vi "Keyence_VS150.vi"(9 "Setting Value":string, 10 "Row No.":string, 11 "Coulumn No.":string) -> (3 "Inspection_Result":bool)   [LabVIEW 2024, in "Keyence_VS150.lvlib"]
doc: "This template is for the Queued Message Handler design pattern.\n\nThe Event Handling Loop generates messages based on user interface actions.\n\nThe Message Handling Loop processes messages generated by the Event Handling Loop, or by other messages. The messages are string values, so new messages can be added easily to the Message Cases case structure in the Message Handling Loop. Each message cluster can also provide an optional value for Message Data, which is a variant that can be converted to whatever message-specific data is required."
uses:
  Keyence_VS150.lvlib
  controls/UI Data.ctl
  Settings/support/Camera.ctl
  <userlib>/_OpenG.lib/array/array.llb/Search 1D Array (String)__ogtk.vi
  <vilib>/Utility/error.llb/Error Cluster From Error Code.vi
  <vilib>/ErrorRing/Error Ring.xnode
  Keysight_34461a/support/Message Queue/Message Queue.lvlib
  support/User Event - Stop/User Event - Stop.lvlib
  support/Message Queue/Message Queue.lvlib
  <userlib>/_OpenG.lib/string/string.llb/openg_string.lvlib
  Launcher/Launcher_DTU.lvlib
  <userlib>/_OpenG.lib/array/array.llb/openg_array.lvlib
  Settings/Setting_Screen.lvlib
panel:
  out "Saturation_Values 2":string
  out "transposed array":string[][](array[string])
  out "appended array":string[][](array[string])
  out "Saturation_Values":string[](array[string])
  in  "Row No. 2":string
  in  "Coulumn No. 2":string
  in  "Setting Value 2":string
  in  "Storage 2":string
  in  "Program No 2":string
  out "data 2":string
  out "Get Mode 2":string
  in  "Change_Program":bool
  out "RX/RY":string
  out "RX,RY":string
  out "status":bool
  in  "Trigger":bool
  in  "Total_Result":T1
  out "DTU 2":string[][](array[string])
  out "DTU1":string[][](array[string])
  out "DTU_Failed_Inspections_Array":string[](array[string])
  out "Fail":i32[](array[numeric])
  out "Inspection_names":string[](array[string])
  out "Result_Values":string[](array[string])
  out "DTU_Failed_Inspections":string
  in  "Config":string
  out "queue name 2":string
  out "queue name":string
  in  "ip address":string="169.254.73.187"
  in  "DUT":string
  out "Result Value":string[](array[string])
  out "Array of Strings":string[](array[string])
  out "data out":string
  out "data":string
  out "Get Mode":string
  in  "Program No":string
  in  "Storage":string
  out "Display <Replace Me>":string
  in  "Exit":bool
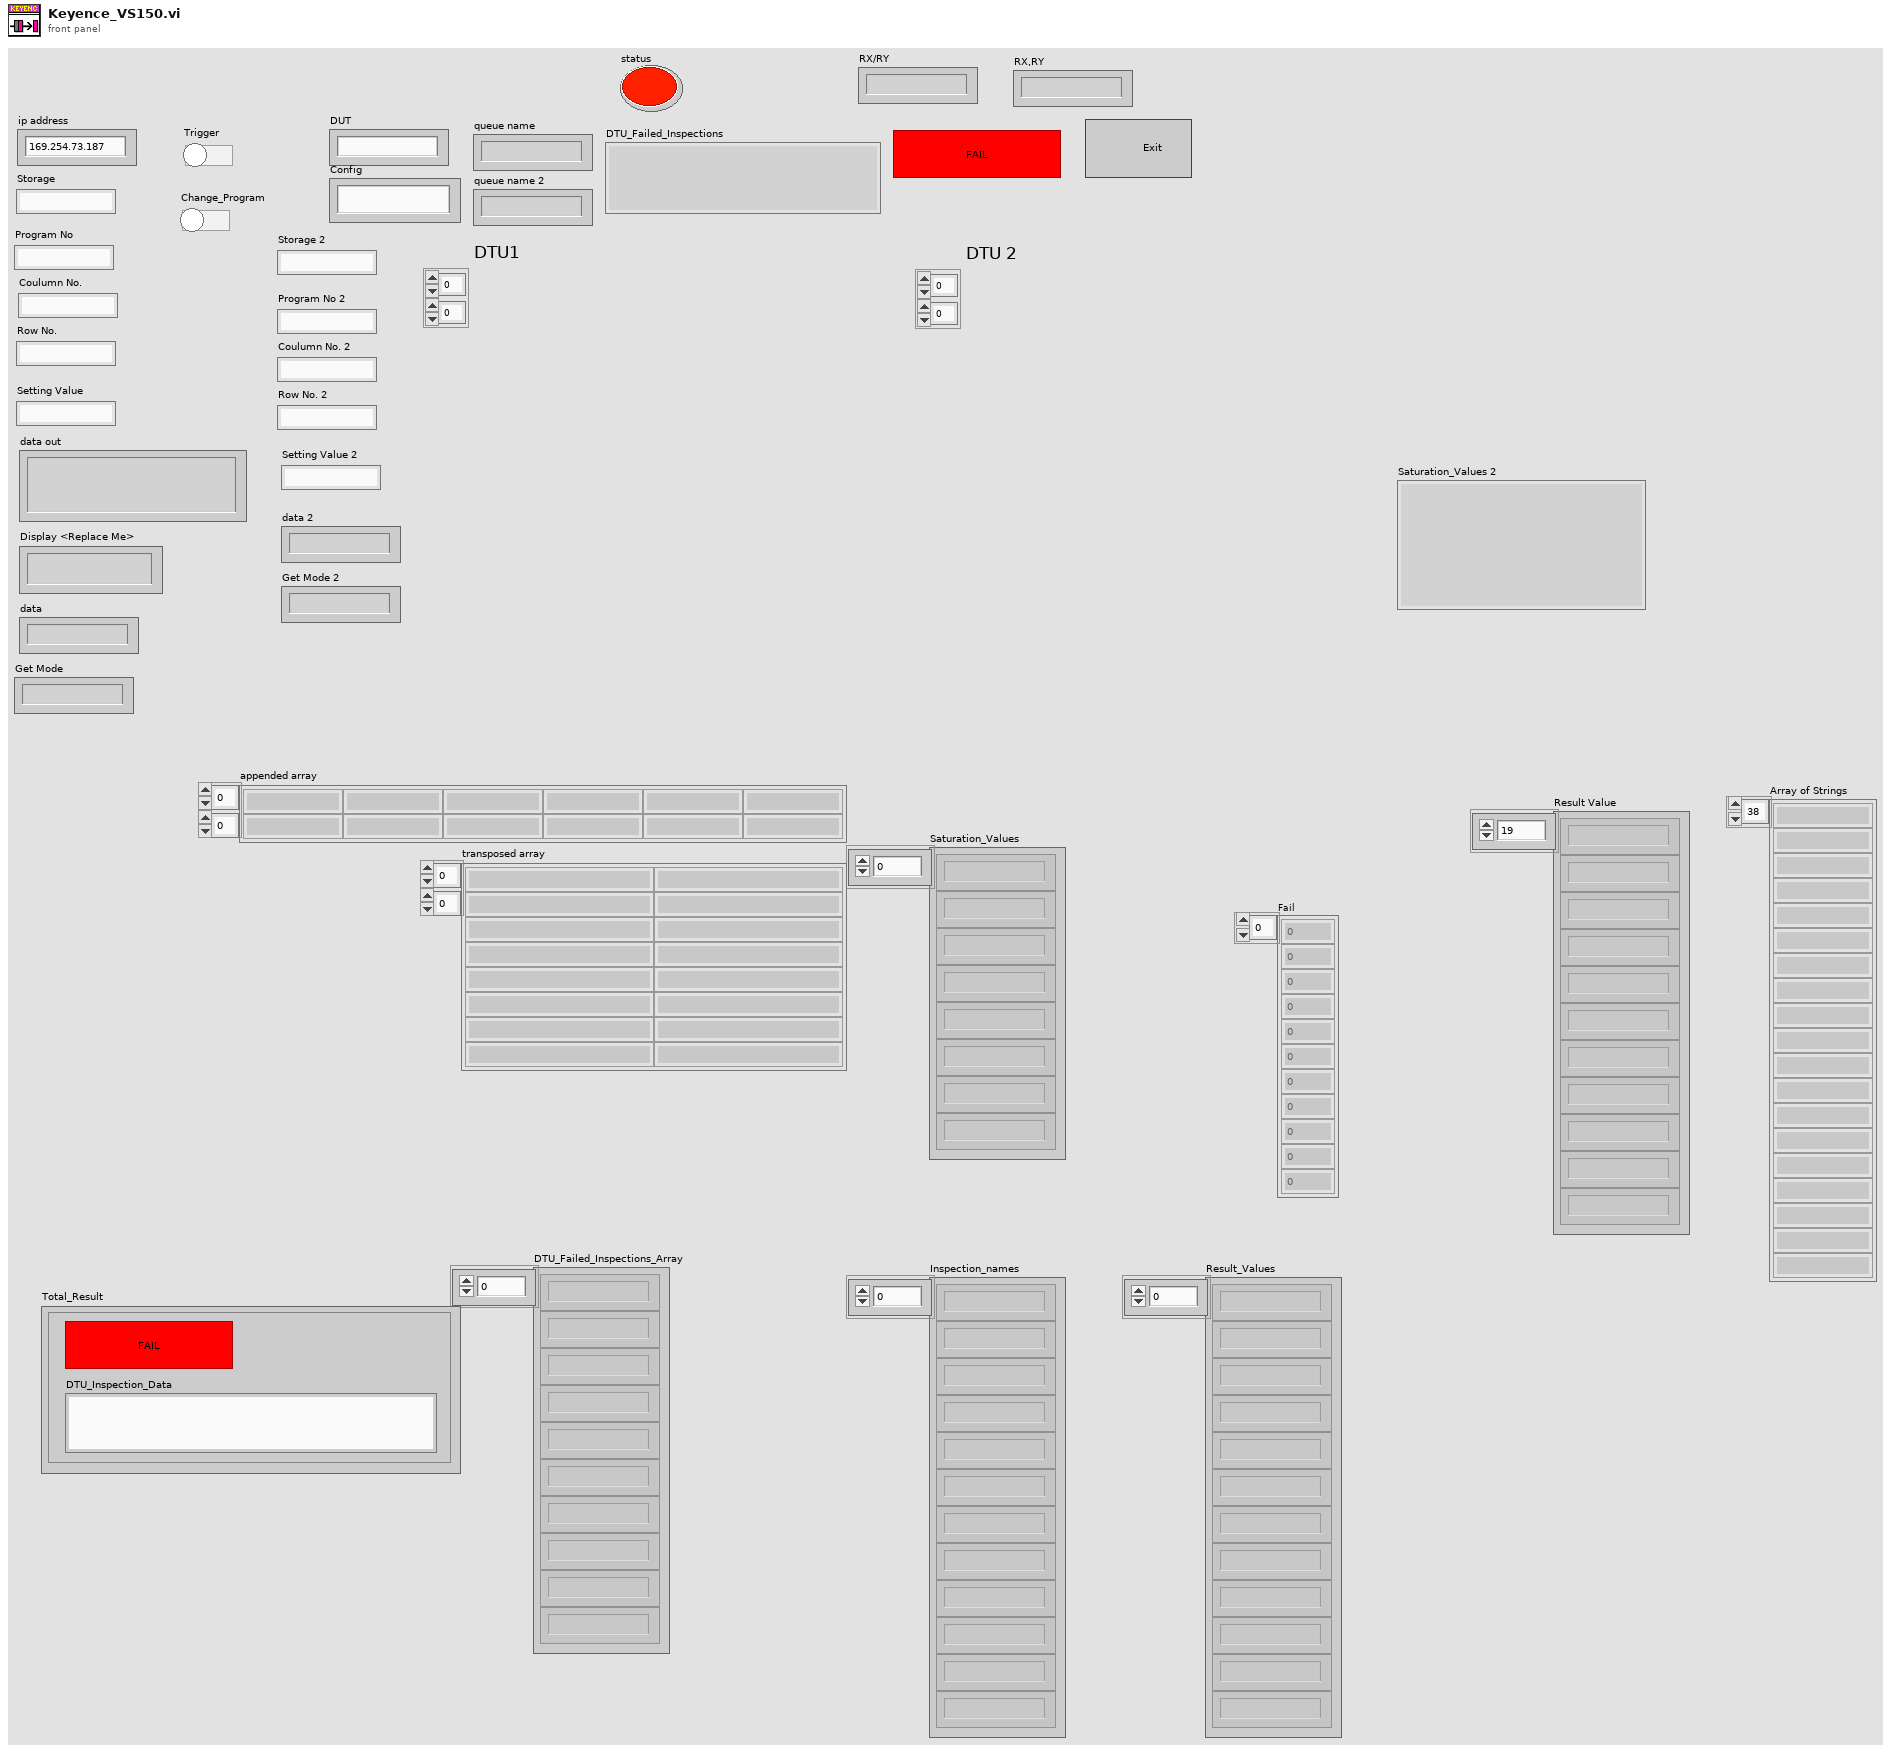
[diagram p1: front panel]
types:
  T1 = cluster{"Inspection_Result 2":bool, "DTU_Inspection_Data":string}
  T2 = typedef "Keyence_VS150.lvlib/UI Data.ctl" = cluster{"Boolean <Replace Me>":bool, "String <Replace Me>":string, "Numeric <Replace Me>":dbl, "Data Display Ref":refnum<vi>, "Exit Button Ref":refnum<vi>, "connection ID":refnum<k5>, "data out":string, "notifier out":refnum<notifier>, "DUT":string, "Config":string, "Keyence_VS150":refnum<queue>, "Result Value":string[], "Inspection_Result":bool, "Total_Result":cluster{"Inspection_Result 2":bool, "Inspection_Data":string}, "Camera":T3, "Camera_Program No":string, "DUT1":string, "DUT2":string, "Saturation_Values":string[]}
  T3 = typedef "Setting_Screen.lvlib/Camera.ctl" = cluster{"Trigger":bool, "Prog No.":string, "Delay":bool, "Delay time":dbl, "Storage":string, "Col no.":string, "Row no.":string}
  T4 = typedef "Keyence_VS150.lvlib/Message Queue.lvlib/All Message Queues.ctl" = cluster{"UI":refnum<queue>, "QSM":refnum<queue>}
  T5 = cluster{"Message":string, "Message Data":variant}
  T6 = enum16{"Read", "Write", "All_sections", "All_values", "Remove key&section"}
  T7 = cluster{"Status":string, "Free/inuse":bool, "Action":string}
  T8 = enum16{"Standard", "Buffered", "CRLF", "Immediate"}
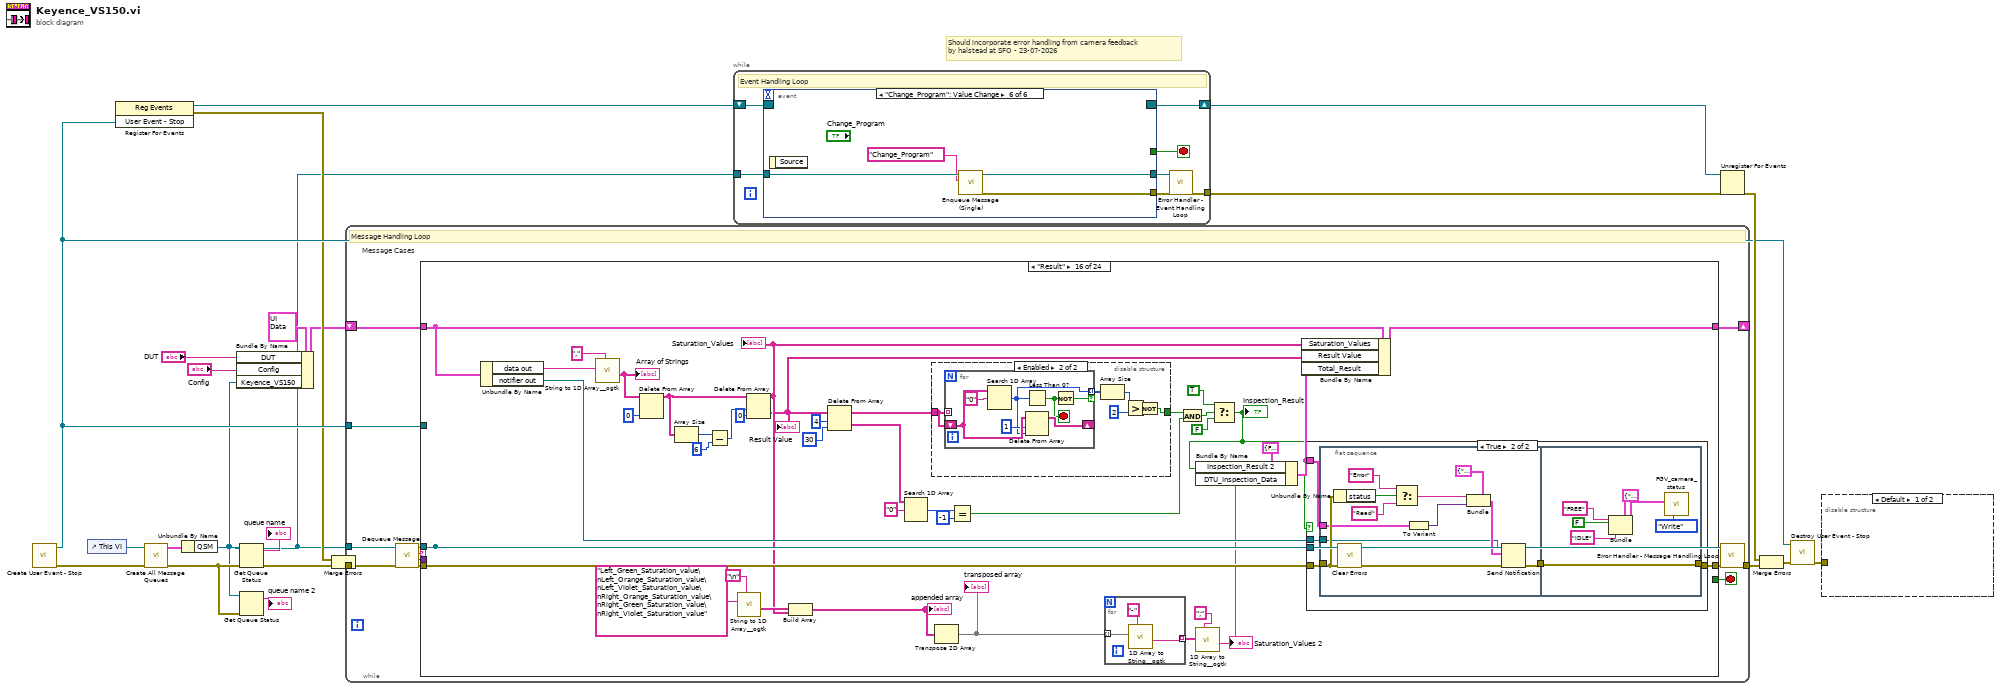
[diagram p0: block diagram]
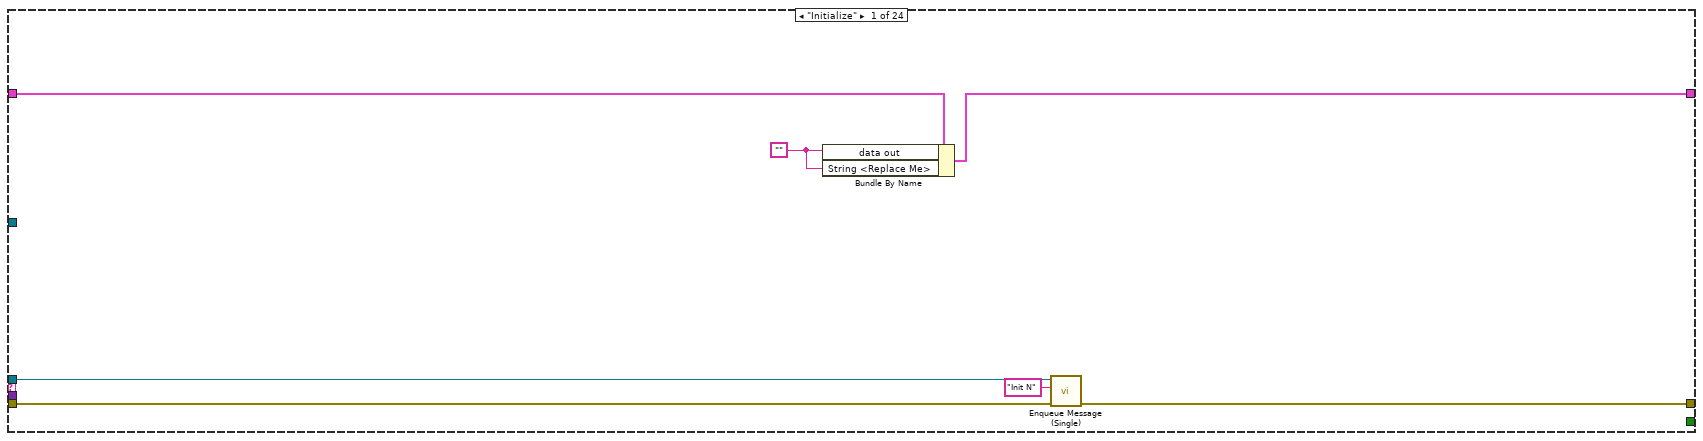
[diagram p2: hidden frame]
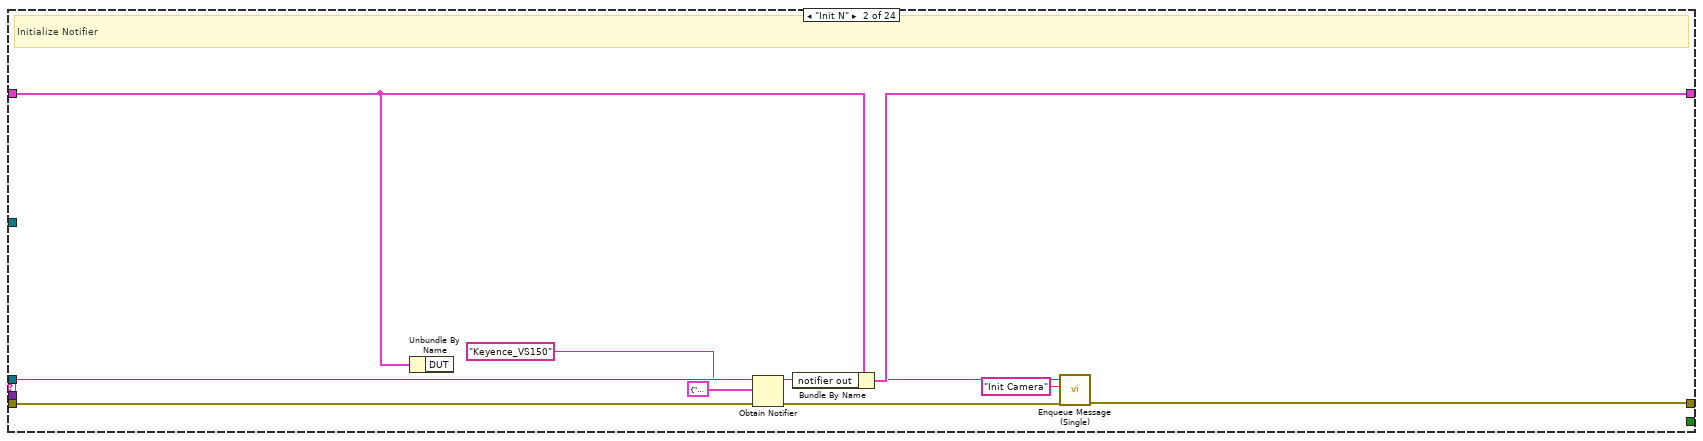
[diagram p3: hidden frame]
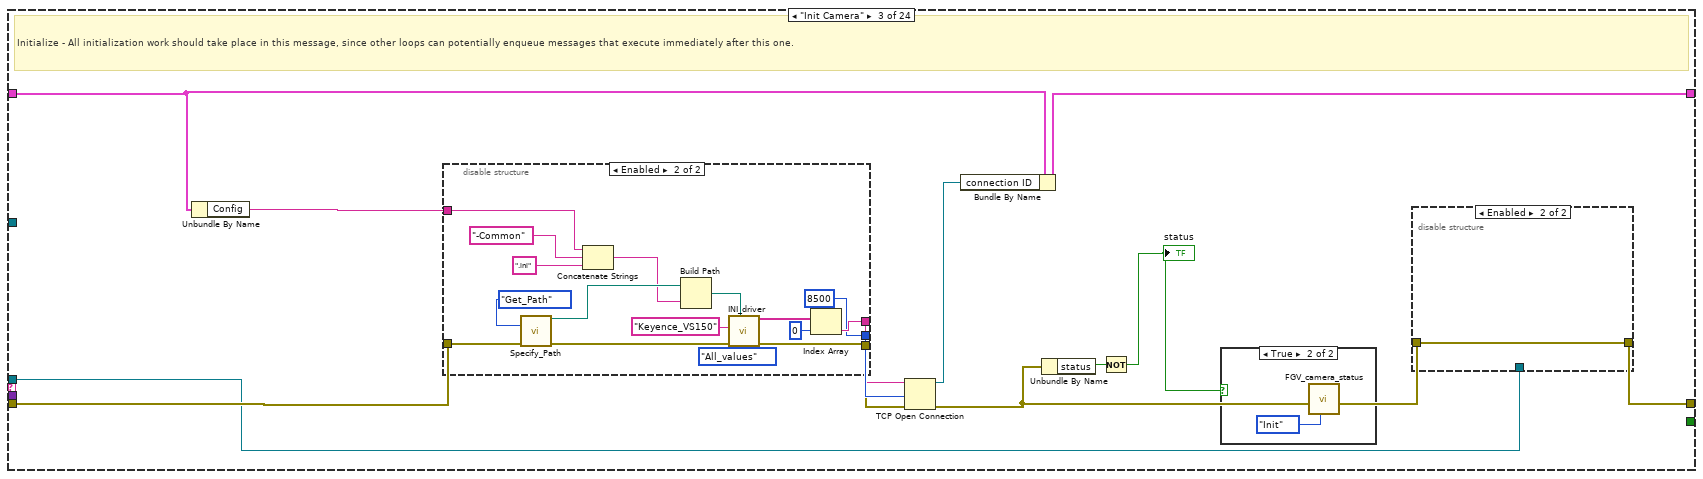
[diagram p4: hidden frame]
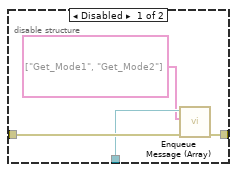
[diagram p5: hidden frame]
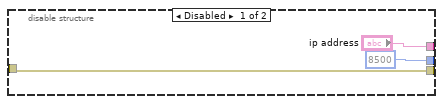
[diagram p7: hidden frame]
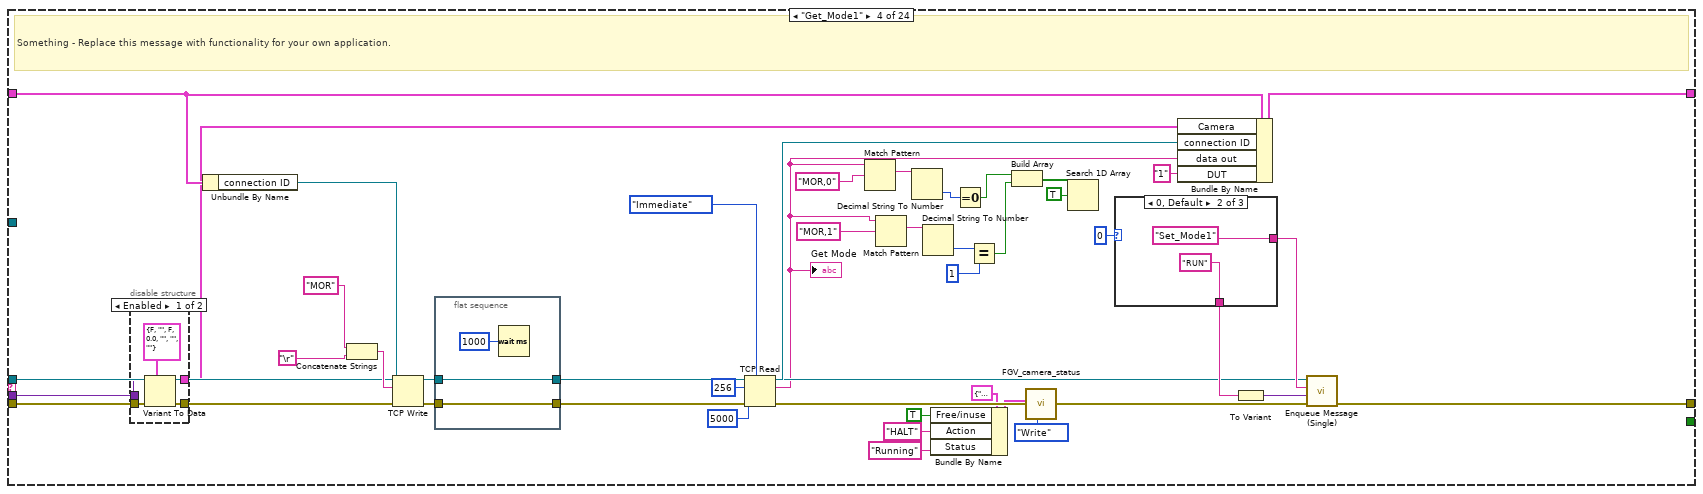
[diagram p8: hidden frame]
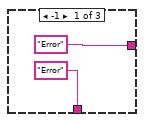
[diagram p10: hidden frame]
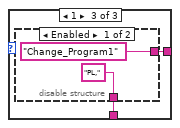
[diagram p11: hidden frame]
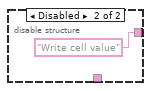
[diagram p12: hidden frame]
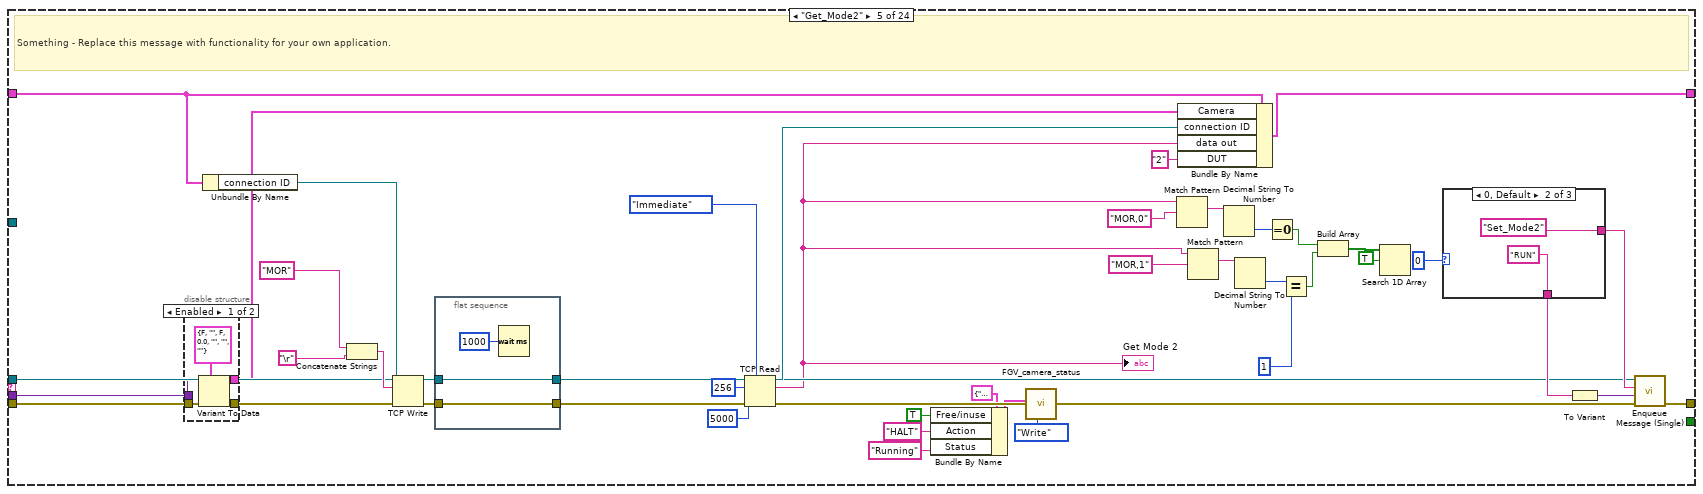
[diagram p13: hidden frame]
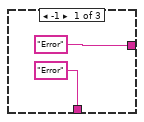
[diagram p15: hidden frame]
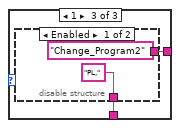
[diagram p16: hidden frame]
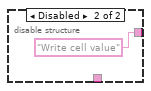
[diagram p17: hidden frame]
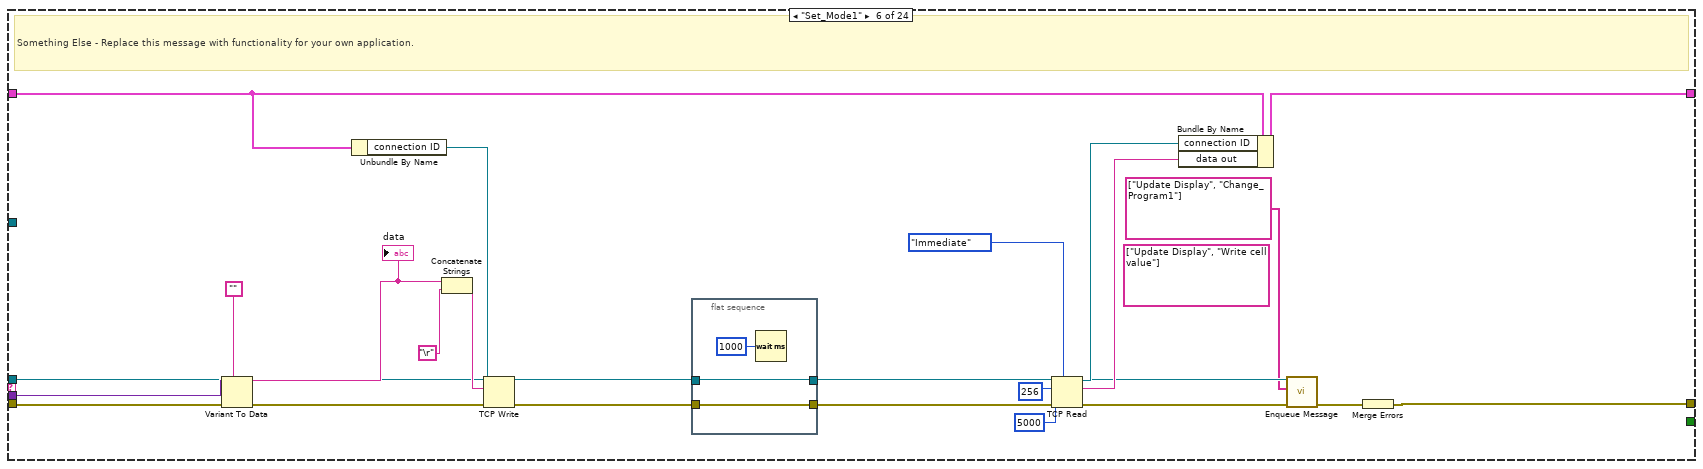
[diagram p18: hidden frame]
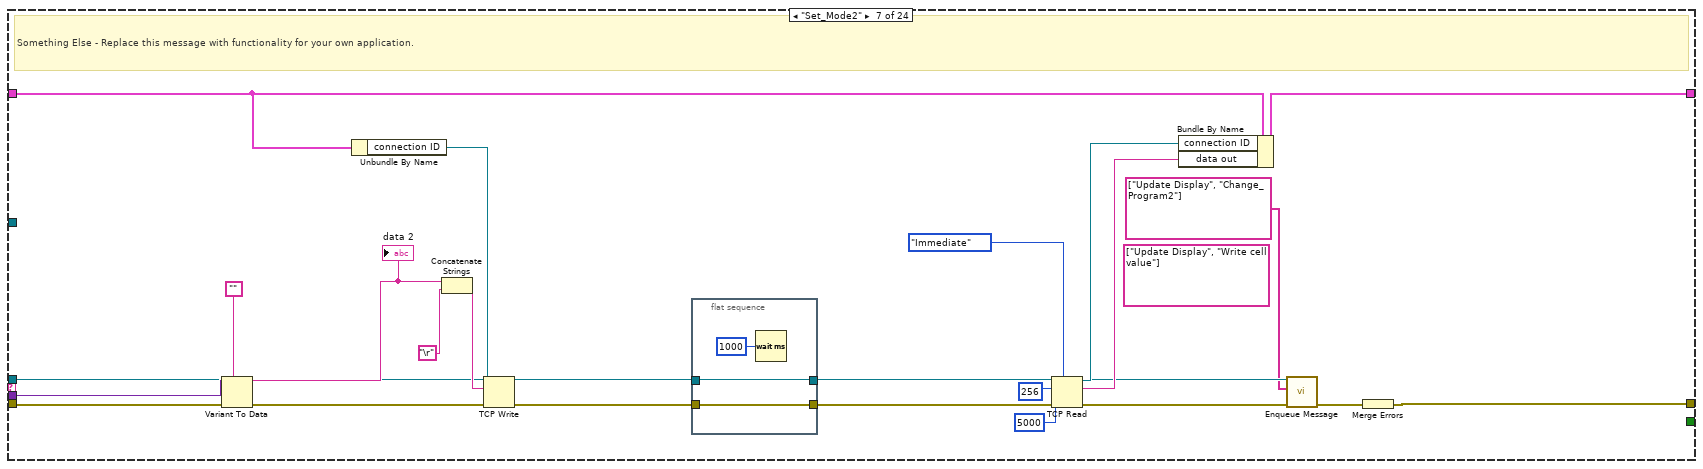
[diagram p19: hidden frame]
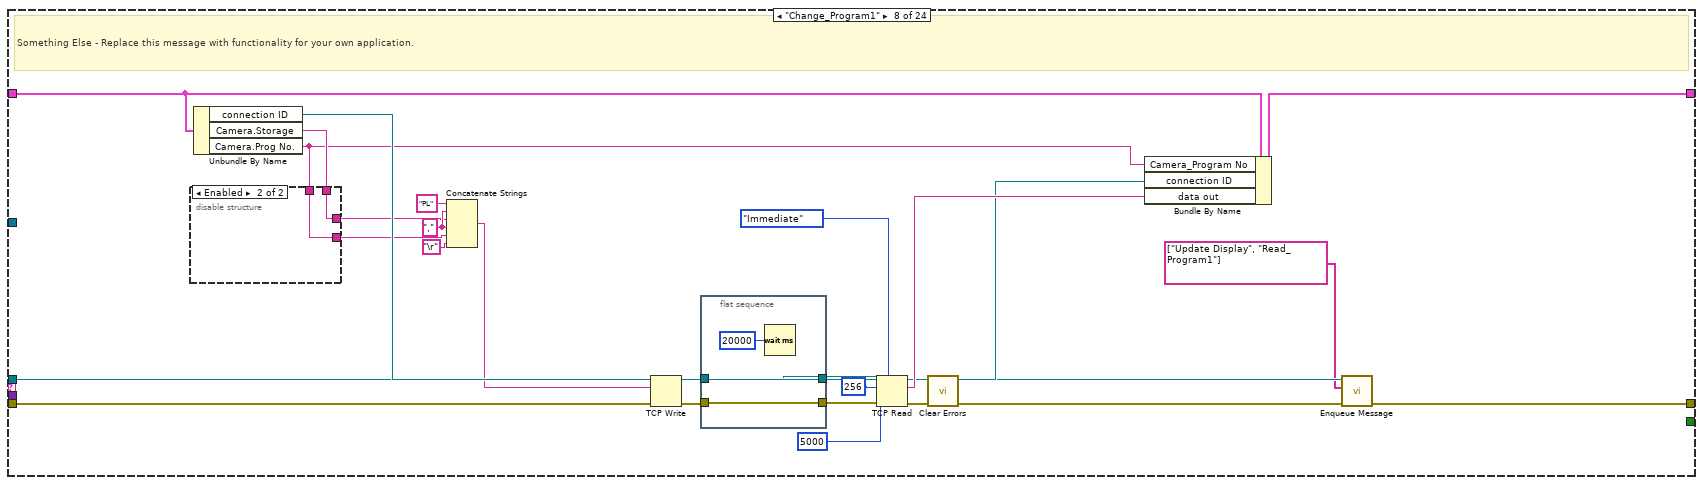
[diagram p20: hidden frame]
diagram:
  # "Should incorporate error handling from camera feedback\nby halstead at SFO - 23-07-2026"
  n1 = call "Create User Event - Stop.vi"() -> ("error out"=w21:errorcluster, "User Event - Stop"=w14:refnum<user-event>)  [unwired: 10 in]
  n2 = control-ref of="This VI"() -> (w9:refnum<vi>)
  n3 = register-events(w14) -> (reference out=w15:refnum<event-registration>, error out=w12:errorcluster)  [unwired: 2 in]
  n4 = call "Create All Message Queues.vi"("error in (no error)"=w21, "This VI"=w9) -> ("error out"=w3:errorcluster, "Message Queues out"=w23:T4)  [unwired: 8 in]
  n5 = Unbundle By Name(w23) -> ("QSM"=w1:refnum<queue>)
  n6 = Bundle By Name(cluster=T2 {"Boolean <Replace Me>"=FALSE, "String <Replace Me>"="", "Numeric <Replace Me>"=0.0, "Data Display Ref"=refnum, "Exit Button Ref"=refnum, "connection ID"=refnum, "data out"="", "notifier out"=refnum, "DUT"="", "Config"="", "Keyence_VS150"=refnum, "Result Value"=[], "Inspection_Result"=FALSE, "Total_Result"={"Inspection_Result 2"=FALSE, "Inspection_Data"=""}, "Camera"={"Trigger"=FALSE, "Prog No."="", "Delay"=FALSE, "Delay time"=0.0, "Storage"="", "Col no."="", "Row no."=""}, "Camera_Program No"="", "DUT1"="", "DUT2"="", "Saturation_Values"=[]} ("Data Cluster"), "DUT"="DUT", "Config"="Config", "Keyence_VS150"=w1) -> (w10:T2)
  n7 = Get Queue Status(queue=w1, error in (no error)=w3) -> (queue out=w5:refnum<queue>, queue name=→"queue name":string, error out=w4:errorcluster)  [unwired: 1 in, 5 out]
  n8 = Get Queue Status(queue=w1, error in (no error)=w3) -> (queue name=→"queue name 2":string)  [unwired: 1 in, 7 out]
  n9 = Merge Errors(w12, w4) -> (w13:errorcluster)
  n10 = while {
    tunnel: w5 -> [w27]
    shift-right: [w34] -> _
    shift-left: w10 -> [w35]
    tunnel: w14 -> [w32]
    tunnel: w13 -> [w31]
    tunnel: [w25] -> w22
    stop <- w33 stop-if-true
    # "Message Handling Loop"
    n11 = call "Dequeue Message.vi"("error in (no error)"=w31, "Message Queue"=w27) -> ("error out"=w30:errorcluster, "Message Data"=w28:variant, "Message"=w29:string, "dup Message Queue"=w26:refnum<queue>)  [unwired: 6 in]
    n12 = case "Message Cases" shown="\"Result\"" w29 {
      selector: w29 -> [_ _ _ _ _ _ _ _ _ _ _ _ _ _ _ _ _ _ _ _ _ _ _ w847]
      tunnel: w26 -> [w37 w45 w54 w116 w177 w219 w246 w284 w317 w338 w385 w452 w503 w547 w575 w637 _ _ _ _ _ w830 w846 _]
      tunnel: w30 -> [w39 w51 w60 w131 w192 w229 w256 w285 w318 w339 w386 w446 w497 w540 w568 w629 w706 w779 w807 w817 w822 w825 w838 _]
      tunnel: [w38 w47 w53 w102 w163 w236 w263 w292 w325 w344 w391 w453 w504 w549 w557 w639 w713 w778 w808 w811 w820 w831 w843 w848] -> w24
      tunnel: w35 -> [w42 w44 w59 w123 w184 w223 w250 w289 w322 w335 w382 w443 w494 w537 w566 w641 w712 w782 w806 w816 w821 w823 w837 w849]
      tunnel: [w40 w49 w64 w122 w183 w222 w249 w288 w321 w341 w388 w442 w493 w536 w565 w640 w712 w782 w806 w816 w821 w823 w837 w849] -> w34
      tunnel: [_ _ _ _ _ _ _ _ _ _ _ _ _ _ _ _ _ _ _ _ _ _ TRUE _] -> w33
      tunnel: w28 -> [_ _ _ w100 w161 w226 w253 _ _ _ _ _ _ _ _ _ _ _ _ w815 _ _ w839 _]
      tunnel: w32 -> [_ _ _ _ _ _ _ _ _ _ _ _ _ _ _ _ _ _ _ _ _ _ w842 _]
      frame "Initialize" {
        w41 = "" ("data out")
        n13 = Bundle By Name(cluster=w42, "data out"=w41, "String <Replace Me>"=w41) -> (w40:T2)
        n14 = call "Enqueue Message (Single).vi"("error in (no error)"=w39, "Message"="Init N", "Message Queue"=w37) -> ("error out"=w38:errorcluster)  [unwired: 7 in, 1 out]
      }
      frame "Init N" {
        # "Initialize Notifier"
        n15 = Unbundle By Name(w44) -> ()  [unwired: 1 out]
        n16 = Obtain Notifier(name (unnamed)="Keyence_VS150", notification data type=T5 {"Message"="", "Message Data"=variant} ("notification"), error in (no error)=w51) -> (notifier out=w50:refnum<notifier>, error out=w48:errorcluster)  [unwired: 1 in, 1 out]
        n17 = Bundle By Name(cluster=w44, "notifier out"=w50) -> (w49:T2)
        n18 = call "Enqueue Message (Single).vi"("error in (no error)"=w48, "Message"="Init Camera", "Message Queue"=w45) -> ("error out"=w47:errorcluster)  [unwired: 7 in, 1 out]
      }
      frame "Init Camera" {
        # "Initialize - All initialization work should take place in this message, since other loops can potentially enqueue messages that execute immediately after this one."
        n19 = Unbundle By Name(w59) -> ("Config"=w58:string)
        n20 = disable-structure shown="Enabled" {
          disable-tunnel: [u16 8500 ("remote port or service name") u16 8500 ("remote port or service name")] -> w65
          disable-tunnel: ["ip address" w77] -> w62
          disable-tunnel: [w72 w78] -> w61
          disable-tunnel: w60 -> [w72 w79]
          disable-tunnel: w58 -> [_ w76]
          frame Disabled {
          }
          frame Enabled {
            n21 = call "Specify_Path.vi"("Path_Enum"=enum16{"Find_Path", "Get_Path"}."Get_Path", "error in (no error)"=w79) -> ("Configurations"=w89:path, "error out"=w86:errorcluster)  [unwired: 6 in, 6 out]
            n22 = Concatenate Strings(w76, "-Common" ("string"), ".ini" ("string")) -> (w81:string)
            n23 = Build Path(base path=w89, name or relative path=w81) -> (appended path=w88:path)
            n24 = call "INI_driver.vi"("Enum"=T6."All_values", "instrument file path"=w88, "error in (no error)"=w86, "Section"="Keyence_VS150") -> ("error out"=w78:errorcluster, "Values out"=w84:string[])  [unwired: 4 in, 2 out]
            n25 = Index Array(array=w84, index=0) -> (element=w77:string)
          }
        }
        n26 = TCP Open Connection(address=w62, remote port or service name=w65, error in (no error)=w61) -> (connection ID=w63:refnum<k5>, error out=w55:errorcluster)  [unwired: 2 in]
        n27 = Bundle By Name(cluster=w59, "connection ID"=w63) -> (w64:T2)
        n28 = Unbundle By Name(w55) -> ("status"=w57:bool)
        n29 = Not(x=w57) -> (.not. x?=w56:bool)
        "status" <- w56
        n30 = case shown="True" w56 {
          frame False {
          }
          frame True {
            n31 = call "FGV_camera_status.vi"("Enum"=enum16{"Init", "Read", "Write"}."Init") -> ()  [unwired: 10 in, 1 out]
          }
        }
        n32 = disable-structure shown="Enabled" {
          disable-tunnel: w55 -> [w69 w70]
          disable-tunnel: w54 -> [w68 _]
          disable-tunnel: [w66 w70] -> w53
          frame Disabled {
            n33 = call "Enqueue Message (Array).vi"("error in (no error)"=w69, "Message Array"=string[] ["Get_Mode1", "Get_Mode2"], "Message Queue"=w68) -> ("error out"=w66:errorcluster)  [unwired: 7 in, 1 out]
          }
          frame Enabled {
          }
        }
      }
      frame "Get_Mode1" {
        # "Something - Replace this message with functionality for your own application."
        n34 = disable-structure shown="Enabled" {
          disable-tunnel: w131 -> [w139 _]
          disable-tunnel: [w138 _] -> w101
          disable-tunnel: w100 -> [w137 _]
          disable-tunnel: [w135 _] -> w99
          frame Enabled {
            n35 = Variant To Data(error in=w139, type=T3 {"Trigger"=FALSE, "Prog No."="", "Delay"=FALSE, "Delay time"=0.0, "Storage"="", "Col no."="", "Row no."=""} ("Camera"), Variant=w137) -> (data=w135:T3, error out=w138:errorcluster)
          }
          frame Disabled {
          }
        }
        n36 = Unbundle By Name(w123) -> ("connection ID"=w124:refnum<k5>)
        n37 = Concatenate Strings("MOR" ("data in"), "\r") -> (w132:string)
        n38 = TCP Write(connection ID=w124, data in=w132, error in (no error)=w101) -> (connection ID out=w118:refnum<k5>, error out=w115:errorcluster)  [unwired: 1 in, 1 out]
        n39 = flat-sequence {
          tunnel: w118 -> [w142]
          tunnel: [w142] -> w117
          tunnel: w115 -> [w140]
          tunnel: [w140] -> w114
          frame #0 {
            n40 = Wait (ms)(milliseconds to wait=u32 1000) -> ()  [unwired: 1 out]
          }
        }
        n41 = TCP Read(connection ID=w117, bytes to read=256, error in (no error)=w114, 7:T8."Immediate" ("mode (standard)"), 9:5000 ("timeout ms (25000)")) -> (connection ID out=w121:refnum<k5>, data out=w110:string, error out=w127:errorcluster)
        "Get Mode" <- w110
        n42 = Match Pattern(string=w110, regular expression="MOR,0") -> (match substring=w112:string)  [unwired: 1 in, 3 out]
        n43 = Match Pattern(string=w110, regular expression="MOR,1") -> (match substring=w111:string)  [unwired: 1 in, 3 out]
        n44 = Decimal String To Number(string=w112) -> (number=w108:i32)  [unwired: 2 in, 1 out]
        n45 = Decimal String To Number(string=w111) -> (number=w106:i32)  [unwired: 2 in, 1 out]
        n46 = Bundle By Name(cluster=T7 {"Status"="", "Free/inuse"=FALSE, "Action"=""} ("Write"), "Free/inuse"=TRUE, "Action"="HALT", "Status"="Running") -> (w95:T7)
        n47 = Equal To 0?(x=w108) -> (x = 0?=w107:bool)
        n48 = Equal?(x=w106, y=1) -> (x = y?=w104:bool)
        n49 = Build Array(w107, w104) -> (w126:bool[])
        n50 = call "FGV_camera_status.vi"("Enum"=enum16{"Init", "Read", "Write"}."Write", "Write"=w95) -> ()  [unwired: 9 in, 1 out]
        n51 = Search 1D Array(1D array=w126, element=TRUE) -> ()  [unwired: 1 in, 1 out]
        n52 = case shown="0, Default" 0 ("index of element") {
          tunnel: ["Error" "Set_Mode1" w148] -> w125
          tunnel: ["Error" "RUN" w147] -> w120
          frame -1 {
          }
          frame 0, Default {
          }
          frame 1 {
            n53 = disable-structure shown="Enabled" {
              disable-tunnel: ["Change_Program1" "Write cell value"] -> w148
              disable-tunnel: ["PL," _] -> w147
              frame Enabled {
              }
              frame Disabled {
              }
            }
          }
        }
        n54 = Bundle By Name(cluster=w123, "Camera"=w99, "connection ID"=w121, "data out"=w110, "DUT"="1" ("DUT1")) -> (w122:T2)
        n55 = To Variant(anything=w120) -> (Variant=w119:variant)
        n56 = call "Enqueue Message (Single).vi"("error in (no error)"=w127, "Message Data"=w119, "Message"=w125, "Message Queue"=w116) -> ("error out"=w102:errorcluster)  [unwired: 6 in, 1 out]
      }
      frame "Get_Mode2" {
        # "Something - Replace this message with functionality for your own application."
        n57 = disable-structure shown="Enabled" {
          disable-tunnel: w192 -> [w200 _]
          disable-tunnel: [w199 _] -> w162
          disable-tunnel: w161 -> [w198 _]
          disable-tunnel: [w197 _] -> w160
          frame Enabled {
            n58 = Variant To Data(error in=w200, type=T3 {"Trigger"=FALSE, "Prog No."="", "Delay"=FALSE, "Delay time"=0.0, "Storage"="", "Col no."="", "Row no."=""} ("Camera"), Variant=w198) -> (data=w197:T3, error out=w199:errorcluster)
          }
          frame Disabled {
          }
        }
        n59 = Unbundle By Name(w184) -> ("connection ID"=w185:refnum<k5>)
        n60 = Concatenate Strings("MOR" ("data in"), "\r") -> (w193:string)
        n61 = TCP Write(connection ID=w185, data in=w193, error in (no error)=w162) -> (connection ID out=w179:refnum<k5>, error out=w176:errorcluster)  [unwired: 1 in, 1 out]
        n62 = flat-sequence {
          tunnel: w179 -> [w203]
          tunnel: [w203] -> w178
          tunnel: w176 -> [w201]
          tunnel: [w201] -> w175
          frame #0 {
            n63 = Wait (ms)(milliseconds to wait=u32 1000) -> ()  [unwired: 1 out]
          }
        }
        n64 = TCP Read(connection ID=w178, bytes to read=256, error in (no error)=w175, 7:T8."Immediate" ("mode (standard)"), 9:5000 ("timeout ms (25000)")) -> (connection ID out=w182:refnum<k5>, data out=w171:string, error out=w188:errorcluster)
        "Get Mode 2" <- w171
        n65 = Bundle By Name(cluster=T7 {"Status"="", "Free/inuse"=FALSE, "Action"=""} ("Write"), "Free/inuse"=TRUE, "Action"="HALT", "Status"="Running") -> (w156:T7)
        n66 = call "FGV_camera_status.vi"("Enum"=enum16{"Init", "Read", "Write"}."Write", "Write"=w156) -> ()  [unwired: 9 in, 1 out]
        n67 = Match Pattern(string=w171, regular expression="MOR,0") -> (match substring=w173:string)  [unwired: 1 in, 3 out]
        n68 = Bundle By Name(cluster=w184, "Camera"=w160, "connection ID"=w182, "data out"=w171, "DUT"="2" ("DUT1")) -> (w183:T2)
        n69 = Match Pattern(string=w171, regular expression="MOR,1") -> (match substring=w172:string)  [unwired: 1 in, 3 out]
        n70 = Decimal String To Number(string=w173) -> (number=w169:i32)  [unwired: 2 in, 1 out]
        n71 = Decimal String To Number(string=w172) -> (number=w167:i32)  [unwired: 2 in, 1 out]
        n72 = Equal To 0?(x=w169) -> (x = 0?=w168:bool)
        n73 = Equal?(x=w167, y=1) -> (x = y?=w165:bool)
        n74 = Build Array(w168, w165) -> (w187:bool[])
        n75 = Search 1D Array(1D array=w187, element=TRUE) -> ()  [unwired: 1 in, 1 out]
        n76 = case shown="0, Default" 0 ("index of element") {
          tunnel: ["Error" "Set_Mode2" w209] -> w186
          tunnel: ["Error" "RUN" w208] -> w181
          frame -1 {
          }
          frame 0, Default {
          }
          frame 1 {
            n77 = disable-structure shown="Enabled" {
              disable-tunnel: ["Change_Program2" "Write cell value"] -> w209
              disable-tunnel: ["PL," _] -> w208
              frame Enabled {
              }
              frame Disabled {
              }
            }
          }
        }
        n78 = To Variant(anything=w181) -> (Variant=w180:variant)
        n79 = call "Enqueue Message (Single).vi"("error in (no error)"=w188, "Message Data"=w180, "Message"=w186, "Message Queue"=w177) -> ("error out"=w163:errorcluster)  [unwired: 6 in, 1 out]
      }
      frame "Set_Mode1" {
        (unwired) string[] ["Update Display", "Write cell value"]
        # "Something Else - Replace this message with functionality for your own application."
        n80 = Variant To Data(error in=w229, type="", Variant=w226) -> (data=w225:string, error out=w228:errorcluster)
        "data" <- w225
        n81 = Unbundle By Name(w223) -> ("connection ID"=w214:refnum<k5>)
        n82 = Concatenate Strings(w225, "\r") -> (w233:string)
        n83 = TCP Write(connection ID=w214, data in=w233, error in (no error)=w228) -> (connection ID out=w216:refnum<k5>, error out=w218:errorcluster)  [unwired: 1 in, 1 out]
        n84 = flat-sequence {
          tunnel: w218 -> [w238]
          tunnel: [w238] -> w217
          tunnel: w216 -> [w237]
          tunnel: [w237] -> w215
          frame #0 {
            n85 = Wait (ms)(milliseconds to wait=u32 1000) -> ()  [unwired: 1 out]
          }
        }
        n86 = TCP Read(connection ID=w215, bytes to read=256, error in (no error)=w217, 7:T8."Immediate" ("mode (standard)"), 9:5000 ("timeout ms (25000)")) -> (connection ID out=w221:refnum<k5>, data out=w220:string, error out=w224:errorcluster)
        n87 = Bundle By Name(cluster=w223, "connection ID"=w221, "data out"=w220) -> (w222:T2)
        n88 = call-poly "Enqueue Message.vi"("error in (no error)"=w224, "Message Array"=string[] ["Update Display", "Change_Program1"], "Message Queue"=w219) -> ("error out"=w235:errorcluster)  [unwired: 7 in, 1 out]
        n89 = Merge Errors(w235) -> (w236:errorcluster)
      }
      frame "Set_Mode2" {
        (unwired) string[] ["Update Display", "Write cell value"]
        # "Something Else - Replace this message with functionality for your own application."
        n90 = Variant To Data(error in=w256, type="", Variant=w253) -> (data=w252:string, error out=w255:errorcluster)
        "data 2" <- w252
        n91 = Unbundle By Name(w250) -> ("connection ID"=w241:refnum<k5>)
        n92 = Concatenate Strings(w252, "\r") -> (w260:string)
        n93 = TCP Write(connection ID=w241, data in=w260, error in (no error)=w255) -> (connection ID out=w243:refnum<k5>, error out=w245:errorcluster)  [unwired: 1 in, 1 out]
        n94 = flat-sequence {
          tunnel: w245 -> [w265]
          tunnel: [w265] -> w244
          tunnel: w243 -> [w264]
          tunnel: [w264] -> w242
          frame #0 {
            n95 = Wait (ms)(milliseconds to wait=u32 1000) -> ()  [unwired: 1 out]
          }
        }
        n96 = TCP Read(connection ID=w242, bytes to read=256, error in (no error)=w244, 7:T8."Immediate" ("mode (standard)"), 9:5000 ("timeout ms (25000)")) -> (connection ID out=w248:refnum<k5>, data out=w247:string, error out=w251:errorcluster)
        n97 = Bundle By Name(cluster=w250, "connection ID"=w248, "data out"=w247) -> (w249:T2)
        n98 = call-poly "Enqueue Message.vi"("error in (no error)"=w251, "Message Array"=string[] ["Update Display", "Change_Program2"], "Message Queue"=w246) -> ("error out"=w262:errorcluster)  [unwired: 7 in, 1 out]
        n99 = Merge Errors(w262) -> (w263:errorcluster)
      }
      frame "Change_Program1" {
        w271 = "," ("string")
        # "Something Else - Replace this message with functionality for your own application."
        n100 = Unbundle By Name(w289) -> ("connection ID"=w291:refnum<k5>, "Camera.Storage"=w268:string, "Camera.Prog No."=w267:string)
        n101 = disable-structure shown="Enabled" {
          disable-tunnel: ["Storage" w296] -> w270
          disable-tunnel: ["Program No" w295] -> w269
          disable-tunnel: w268 -> [_ w296]
          disable-tunnel: w267 -> [_ w295]
          frame Disabled {
          }
          frame Enabled {
          }
        }
        n102 = Concatenate Strings("PL" ("string"), w271, w270, w271, w269, "\r") -> (w282:string)
        n103 = TCP Write(connection ID=w291, data in=w282, error in (no error)=w285) -> (connection ID out=w276:refnum<k5>, error out=w275:errorcluster)  [unwired: 1 in, 1 out]
        n104 = flat-sequence {
          tunnel: w276 -> [w299]
          tunnel: [w299] -> w273
          tunnel: w275 -> [w297]
          tunnel: [w297] -> w274
          frame #0 {
            n105 = Wait (ms)(milliseconds to wait=u32 20000) -> ()  [unwired: 1 out]
          }
        }
        n106 = TCP Read(connection ID=w273, bytes to read=256, error in (no error)=w274, 7:T8."Immediate" ("mode (standard)"), 9:5000 ("timeout ms (25000)")) -> (connection ID out=w286:refnum<k5>, data out=w287:string, error out=w277:errorcluster)
        n107 = call <vilib>:"Clear Errors.vi"("error in (no error)"=w277) -> ("error out"=w290:errorcluster)  [unwired: 5 in, 1 out]
        n108 = Bundle By Name(cluster=w289, "Camera_Program No"=w267, "connection ID"=w286, "data out"=w287) -> (w288:T2)
        n109 = call-poly "Enqueue Message.vi"("error in (no error)"=w290, "Message Array"=string[] ["Update Display", "Read_Program1"], "Message Queue"=w284) -> ("error out"=w292:errorcluster)  [unwired: 7 in, 1 out]
      }
      frame "Change_Program2" {
        w304 = "," ("string")
        # "Something Else - Replace this message with functionality for your own application."
        n110 = Unbundle By Name(w322) -> ("connection ID"=w324:refnum<k5>, "Camera.Storage"=w301:string, "Camera.Prog No."=w300:string)
        n111 = disable-structure shown="Enabled" {
          disable-tunnel: ["Storage 2" w329] -> w303
          disable-tunnel: ["Program No 2" w328] -> w302
          disable-tunnel: w301 -> [_ w329]
          disable-tunnel: w300 -> [_ w328]
          frame Disabled {
          }
          frame Enabled {
          }
        }
        n112 = Concatenate Strings("PL" ("string"), w304, w303, w304, w302, "\r") -> (w315:string)
        n113 = TCP Write(connection ID=w324, data in=w315, error in (no error)=w318) -> (connection ID out=w309:refnum<k5>, error out=w308:errorcluster)  [unwired: 1 in, 1 out]
        n114 = flat-sequence {
          tunnel: w309 -> [w332]
          tunnel: [w332] -> w306
          tunnel: w308 -> [w330]
          tunnel: [w330] -> w307
          frame #0 {
            n115 = Wait (ms)(milliseconds to wait=u32 20000) -> ()  [unwired: 1 out]
          }
        }
        n116 = TCP Read(connection ID=w306, bytes to read=256, error in (no error)=w307, 7:T8."Immediate" ("mode (standard)"), 9:5000 ("timeout ms (25000)")) -> (connection ID out=w319:refnum<k5>, data out=w320:string, error out=w310:errorcluster)
        n117 = call <vilib>:"Clear Errors.vi"("error in (no error)"=w310) -> ("error out"=w323:errorcluster)  [unwired: 5 in, 1 out]
        n118 = Bundle By Name(cluster=w322, "Camera_Program No"=w300, "connection ID"=w319, "data out"=w320) -> (w321:T2)
        n119 = call-poly "Enqueue Message.vi"("error in (no error)"=w323, "Message Array"=string[] ["Update Display", "Read_Program2"], "Message Queue"=w317) -> ("error out"=w325:errorcluster)  [unwired: 7 in, 1 out]
      }
      frame "Read_Program1" {
        # "Something Else - Replace this message with functionality for your own application."
        n120 = Unbundle By Name(w335) -> ("connection ID"=w343:refnum<k5>)
        n121 = Unbundle By Name(w335) -> ("Camera_Program No"=w334:string)
        n122 = for {
          N: 3 -> [_]
          tunnel: [w358] -> w336
          shift-right: [w367] -> w340
          shift-left: w343 -> [w369]
          shift-right: [w357] -> w342
          shift-left: w339 -> [w366]
          tunnel: w334 -> [w353]
          tunnel: [w356] -> w333
          stop <- w356 stop-if-true
          n123 = Concatenate Strings("PR" ("string"), "\r") -> (w374:string)
          n124 = TCP Write(connection ID=w369, data in=w374, error in (no error)=w366) -> (connection ID out=w365:refnum<k5>, error out=w364:errorcluster)  [unwired: 1 in, 1 out]
          n125 = flat-sequence {
            tunnel: w365 -> [w379]
            tunnel: [w379] -> w362
            tunnel: w364 -> [w377]
            tunnel: [w377] -> w363
            frame #0 {
              n126 = Wait (ms)(milliseconds to wait=u32 1000) -> ()  [unwired: 1 out]
            }
          }
          n127 = disable-structure shown="Enabled" {
            disable-tunnel: [w375 w376] -> w354
            disable-tunnel: w353 -> [_ w376]
            frame Disabled {
              n128 = local read "Program No"() -> (w375:string)
            }
            frame Enabled {
            }
          }
          n129 = TCP Read(connection ID=w362, bytes to read=256, error in (no error)=w363, 7:T8."Immediate" ("mode (standard)"), 9:5000 ("timeout ms (25000)")) -> (connection ID out=w367:refnum<k5>, data out=w358:string, error out=w368:errorcluster)
          n130 = String Subset(string=w358, offset (0)=5, length (rest)=1 ("length (rest)")) -> (substring=w360:string)
          n131 = call <vilib>:"Clear Errors.vi"("error in (no error)"=w368) -> ("error out"=w357:errorcluster)  [unwired: 5 in, 1 out]
          n132 = Equal?(x=w354, y=w360) -> (x = y?=w356:bool)
        }
        n133 = case shown="True" w333 {
          tunnel: [w347 w352] -> w344
          tunnel: w342 -> [w348 w351]
          tunnel: w338 -> [w346 w350]
          frame False {
            n134 = call-poly "Enqueue Message.vi"("error in (no error)"=w348, "Message"="Change_Program1", "Message Queue"=w346) -> ("error out"=w347:errorcluster)  [unwired: 7 in, 1 out]
          }
          frame True {
            n135 = call-poly "Enqueue Message.vi"("error in (no error)"=w351, "Message Array"=string[] ["Update Display", "Write cell value1"], "Message Queue"=w350) -> ("error out"=w352:errorcluster)  [unwired: 7 in, 1 out]
          }
        }
        n136 = Bundle By Name(cluster=w335, "connection ID"=w340, "data out"=w336) -> (w341:T2)
      }
      frame "Read_Program2" {
        # "Something Else - Replace this message with functionality for your own application."
        n137 = Unbundle By Name(w382) -> ("connection ID"=w390:refnum<k5>)
        n138 = Unbundle By Name(w382) -> ("Camera_Program No"=w380:string)
        n139 = for {
          N: 3 -> [_]
          tunnel: [w405] -> w383
          shift-right: [w414] -> w387
          shift-left: w390 -> [w416]
          shift-right: [w404] -> w389
          shift-left: w386 -> [w413]
          tunnel: [w403] -> w381
          tunnel: w380 -> [w401]
          stop <- w403 stop-if-true
          n140 = Concatenate Strings("PR" ("string"), "\r") -> (w421:string)
          n141 = TCP Write(connection ID=w416, data in=w421, error in (no error)=w413) -> (connection ID out=w412:refnum<k5>, error out=w411:errorcluster)  [unwired: 1 in, 1 out]
          n142 = flat-sequence {
            tunnel: w412 -> [w426]
            tunnel: [w426] -> w409
            tunnel: w411 -> [w424]
            tunnel: [w424] -> w410
            frame #0 {
              n143 = Wait (ms)(milliseconds to wait=u32 1000) -> ()  [unwired: 1 out]
            }
          }
          n144 = disable-structure shown="Enabled" {
            disable-tunnel: [w422 w423] -> w400
            disable-tunnel: w401 -> [_ w423]
            frame Disabled {
              n145 = local read "Program No"() -> (w422:string)
            }
            frame Enabled {
            }
          }
          n146 = TCP Read(connection ID=w409, bytes to read=256, error in (no error)=w410, 7:T8."Immediate" ("mode (standard)"), 9:5000 ("timeout ms (25000)")) -> (connection ID out=w414:refnum<k5>, data out=w405:string, error out=w415:errorcluster)
          n147 = String Subset(string=w405, offset (0)=5, length (rest)=1 ("length (rest)")) -> (substring=w407:string)
          n148 = call <vilib>:"Clear Errors.vi"("error in (no error)"=w415) -> ("error out"=w404:errorcluster)  [unwired: 5 in, 1 out]
          n149 = Equal?(x=w400, y=w407) -> (x = y?=w403:bool)
        }
        n150 = case shown="True" w381 {
          tunnel: [w394 w399] -> w391
          tunnel: w389 -> [w395 w398]
          tunnel: w385 -> [w393 w397]
          frame False {
            n151 = call-poly "Enqueue Message.vi"("error in (no error)"=w395, "Message"="Change_Program2", "Message Queue"=w393) -> ("error out"=w394:errorcluster)  [unwired: 7 in, 1 out]
          }
          frame True {
            n152 = call-poly "Enqueue Message.vi"("error in (no error)"=w398, "Message Array"=string[] ["Update Display", "Write cell value2"], "Message Queue"=w397) -> ("error out"=w399:errorcluster)  [unwired: 7 in, 1 out]
          }
        }
        n153 = Bundle By Name(cluster=w382, "connection ID"=w387, "data out"=w383) -> (w388:T2)
      }
      frame "Write cell value1" {
        w439 = "," ("string")
        # "Something Else - Replace this message with functionality for your own application."
        n154 = Unbundle By Name(w443) -> ("notifier out"=w432:refnum<notifier>, "connection ID"=w444:refnum<k5>, "DUT"=w433:string, "Camera.Col no."=w430:string, "Camera.Row no."=w428:string)
        n155 = disable-structure shown="Enabled" {
          disable-tunnel: w430 -> [_ w457]
          disable-tunnel: ["Coulumn No." w457] -> w429
          disable-tunnel: w428 -> [_ w456]
          disable-tunnel: ["Row No." w456] -> w427
          frame Disabled {
          }
          frame Enabled {
          }
        }
        n156 = disable-structure shown="Enabled" {
          disable-tunnel: [w473 "Setting Value"] -> w434
          disable-tunnel: w433 -> [w473 _]
          frame Enabled {
          }
          frame Disabled {
          }
        }
        n157 = Concatenate Strings("CWN," ("data in"), w429, w439, w427, w439, w434, "\r") -> (w451:string)
        n158 = TCP Write(connection ID=w444, data in=w451, error in (no error)=w446) -> (connection ID out=w438:refnum<k5>, error out=w437:errorcluster)  [unwired: 1 in, 1 out]
        n159 = flat-sequence {
          tunnel: w438 -> [w477]
          tunnel: [w477] -> w435
          tunnel: w437 -> [w475]
          tunnel: [w475] -> w436
          frame #0 {
            n160 = Wait (ms)(milliseconds to wait=u32 1000) -> ()  [unwired: 1 out]
          }
        }
        n161 = TCP Read(connection ID=w435, bytes to read=256, error in (no error)=w436, 7:T8."Immediate" ("mode (standard)"), 9:5000 ("timeout ms (25000)")) -> (connection ID out=w440:refnum<k5>, data out=w441:string, error out=w445:errorcluster)
        n162 = disable-structure shown="Enabled" {
          disable-tunnel: [w462 w465] -> w453
          disable-tunnel: w452 -> [w460 _]
          disable-tunnel: w445 -> [w459 w464]
          disable-tunnel: w432 -> [_ w463]
          frame Disabled {
            n163 = call-poly "Enqueue Message.vi"("error in (no error)"=w459, "Message Array"=string[] ["Update Display", "Trigger"], "Message Queue"=w460) -> ("error out"=w461:errorcluster)  [unwired: 7 in, 1 out]
            n164 = Merge Errors(w461) -> (w462:errorcluster)
          }
          frame Enabled {
            n165 = Unbundle By Name(w464) -> ("status"=w472:bool)
            n166 = Select(t="Error" ("f"), s=w472, f="Step_Done" ("Message")) -> (s? t:f=w468:string)
            n167 = Bundle By Name(cluster=T5 {"Message"="", "Message Data"=variant} ("notification"), "Message"=w468) -> (w467:T5)
            n168 = call <vilib>:"Clear Errors.vi"("error in (no error)"=w464) -> ("error out"=w466:errorcluster)  [unwired: 5 in, 1 out]
            n169 = Send Notification(notification=w467, notifier=w463, error in (no error)=w466) -> (error out=w465:errorcluster)  [unwired: 1 out]
          }
        }
        n170 = Bundle By Name(cluster=w443, "connection ID"=w440, "data out"=w441) -> (w442:T2)
      }
      frame "Write cell value2" {
        w489 = "," ("string")
        # "Something Else - Replace this message with functionality for your own application."
        n171 = Unbundle By Name(w494) -> ("notifier out"=w482:refnum<notifier>, "connection ID"=w495:refnum<k5>, "DUT"=w483:string, "Camera.Col no."=w479:string, "Camera.Row no."=w478:string)
        n172 = disable-structure shown="Enabled" {
          disable-tunnel: ["Coulumn No. 2" w508] -> w481
          disable-tunnel: ["Row No. 2" w507] -> w480
          disable-tunnel: w479 -> [_ w508]
          disable-tunnel: w478 -> [_ w507]
          frame Disabled {
          }
          frame Enabled {
          }
        }
        n173 = disable-structure shown="Enabled" {
          disable-tunnel: [w524 "Setting Value 2"] -> w484
          disable-tunnel: w483 -> [w524 _]
          frame Enabled {
          }
          frame Disabled {
          }
        }
        n174 = Concatenate Strings("CWN," ("data in"), w481, w489, w480, w489, w484, "\r") -> (w502:string)
        n175 = TCP Write(connection ID=w495, data in=w502, error in (no error)=w497) -> (connection ID out=w488:refnum<k5>, error out=w487:errorcluster)  [unwired: 1 in, 1 out]
        n176 = flat-sequence {
          tunnel: w488 -> [w528]
          tunnel: [w528] -> w485
          tunnel: w487 -> [w526]
          tunnel: [w526] -> w486
          frame #0 {
            n177 = Wait (ms)(milliseconds to wait=u32 1000) -> ()  [unwired: 1 out]
          }
        }
        n178 = TCP Read(connection ID=w485, bytes to read=256, error in (no error)=w486, 7:T8."Immediate" ("mode (standard)"), 9:5000 ("timeout ms (25000)")) -> (connection ID out=w491:refnum<k5>, data out=w492:string, error out=w496:errorcluster)
        n179 = disable-structure shown="Enabled" {
          disable-tunnel: [w513 w516] -> w504
          disable-tunnel: w503 -> [w511 _]
          disable-tunnel: w496 -> [w510 w515]
          disable-tunnel: w482 -> [_ w514]
          frame Disabled {
            n180 = call-poly "Enqueue Message.vi"("error in (no error)"=w510, "Message Array"=string[] ["Update Display", "Trigger"], "Message Queue"=w511) -> ("error out"=w512:errorcluster)  [unwired: 7 in, 1 out]
            n181 = Merge Errors(w512) -> (w513:errorcluster)
          }
          frame Enabled {
            n182 = Unbundle By Name(w515) -> ("status"=w523:bool)
            n183 = Select(t="Error" ("f"), s=w523, f="Step_Done" ("Message")) -> (s? t:f=w519:string)
            n184 = Bundle By Name(cluster=T5 {"Message"="", "Message Data"=variant} ("notification"), "Message"=w519) -> (w518:T5)
            n185 = call <vilib>:"Clear Errors.vi"("error in (no error)"=w515) -> ("error out"=w517:errorcluster)  [unwired: 5 in, 1 out]
            n186 = Send Notification(notification=w518, notifier=w514, error in (no error)=w517) -> (error out=w516:errorcluster)  [unwired: 1 out]
          }
        }
        n187 = Bundle By Name(cluster=w494, "connection ID"=w491, "data out"=w492) -> (w493:T2)
      }
      frame "Trigger" {
        # "Something Else - Replace this message with functionality for your own application."
        n188 = Unbundle By Name(w537) -> ("connection ID"=w539:refnum<k5>)
        n189 = Concatenate Strings("TRG" ("data in"), "\r") -> (w544:string)
        n190 = TCP Write(connection ID=w539, data in=w544, error in (no error)=w540) -> (connection ID out=w532:refnum<k5>, error out=w531:errorcluster)  [unwired: 1 in, 1 out]
        n191 = flat-sequence {
          tunnel: w532 -> [w552]
          tunnel: [w552] -> w529
          tunnel: w531 -> [w550]
          tunnel: [w550] -> w530
          frame #0 {
            n192 = Wait (ms)(milliseconds to wait=u32 7000) -> ()  [unwired: 1 out]
          }
        }
        n193 = TCP Read(connection ID=w529, bytes to read=256, error in (no error)=w530, 7:T8."Immediate" ("mode (standard)"), 9:5000 ("timeout ms (25000)")) -> (connection ID out=w535:refnum<k5>, data out=w534:string, error out=w538:errorcluster)
        n194 = Bundle By Name(cluster=w537, "connection ID"=w535, "data out"=w534) -> (w536:T2)
        n195 = call "Enqueue Message (Single).vi"("error in (no error)"=w538, "Message"="Trigger2", "Message Queue"=w547) -> ("error out"=w548:errorcluster)  [unwired: 7 in, 1 out]
        n196 = Merge Errors(w548) -> (w549:errorcluster)
      }
      frame "Trigger2" {
        # "Something Else - Replace this message with functionality for your own application."
        n197 = Unbundle By Name(w566) -> ("connection ID"=w567:refnum<k5>, "Camera.Prog No."=w554:string)
        n198 = Concatenate Strings("TRG" ("data in"), "\r") -> (w572:string)
        n199 = TCP Write(connection ID=w567, data in=w572, error in (no error)=w568) -> (connection ID out=w562:refnum<k5>, error out=w561:errorcluster)  [unwired: 1 in, 1 out]
        n200 = flat-sequence {
          tunnel: w562 -> [w605]
          tunnel: [w605] -> w559
          tunnel: w561 -> [w603]
          tunnel: [w603] -> w560
          frame #0 {
            n201 = Wait (ms)(milliseconds to wait=u32 7000) -> ()  [unwired: 1 out]
          }
        }
        n202 = TCP Read(connection ID=w559, bytes to read=256, error in (no error)=w560, 7:T8."Immediate" ("mode (standard)"), 9:5000 ("timeout ms (25000)")) -> (connection ID out=w564:refnum<k5>, data out=w563:string, error out=w558:errorcluster)
        "data out" <- w563
        n203 = disable-structure shown="Enabled" {
          disable-tunnel: w554 -> [_ w577]
          disable-tunnel: [w576 w577] -> w553
          frame Disabled {
            n204 = local read "Program No"() -> (w576:string)
          }
          frame Enabled {
          }
        }
        n205 = Equal?(x=w553, y="5") -> (x = y?=w555:bool)
        n206 = case shown="False" w555 {
          tunnel: w575 -> [w581 w602]
          tunnel: w558 -> [w580 w600]
          tunnel: [w579 w599] -> w557
          tunnel: w553 -> [w578 _]
          frame False {
            n207 = Equal?(x=w578, y="9") -> (x = y?=w582:bool)
            n208 = case shown="True" w582 {
              tunnel: w581 -> [w584 w597]
              tunnel: w580 -> [w587 w596]
              tunnel: [w585 w595] -> w579
              tunnel: w578 -> [w588 _]
              frame False {
                n209 = Equal?(x=w588, y="2") -> (x = y?=w586:bool)
                n210 = case shown="True" w586 {
                  tunnel: w587 -> [w590 w593]
                  tunnel: [w590 w592] -> w585
                  tunnel: w584 -> [_ w591]
                  frame False {
                  }
                  frame True {
                    n211 = call-poly "Enqueue Message.vi"("error in (no error)"=w593, "Message Array"=string[] ["Update Display", "Result"], "Message Queue"=w591) -> ("error out"=w592:errorcluster)  [unwired: 7 in, 1 out]
                  }
                }
              }
              frame True {
                n212 = call-poly "Enqueue Message.vi"("error in (no error)"=w596, "Message Array"=string[] ["Update Display", "Result"], "Message Queue"=w597) -> ("error out"=w595:errorcluster)  [unwired: 7 in, 1 out]
              }
            }
          }
          frame True {
            n213 = call-poly "Enqueue Message.vi"("error in (no error)"=w600, "Message Array"=string[] ["Update Display", "SSL_Result"], "Message Queue"=w602) -> ("error out"=w599:errorcluster)  [unwired: 7 in, 1 out]
          }
        }
        n214 = Bundle By Name(cluster=w566, "connection ID"=w564, "data out"=w563) -> (w565:T2)
      }
      frame "Result" {
        n215 = Unbundle By Name(w641) -> ("data out"=w644:string, "notifier out"=w638:refnum<notifier>)
        n216 = call <userlib>:"String to 1D Array__ogtk.vi"("delimiter (Tab)"=",", "string"=w644) -> ("Array of Strings"=w643:string[])  [unwired: 9 in]
        "Array of Strings" <- w643
        n217 = Delete From Array(array=w643, index=0) -> (array with subset deleted=w633:string[])  [unwired: 1 in, 1 out]
        n218 = Array Size(array=w633) -> (size(s)=w628:i32)
        n219 = Subtract(x=w628, y=6) -> (x-y=w627:i32)
        n220 = call <userlib>:"String to 1D Array__ogtk.vi"("delimiter (Tab)"="\n", "string"="Left_Green_Saturation_value\nLeft_Orange_Saturation_value\nLeft_Violet_Saturation_value\nRight_Orange_Saturation_value\nRight_Green_Saturation_value\nRight_Violet_Saturation_value") -> ("Array of Strings"=w622:string[])  [unwired: 9 in]
        n221 = Delete From Array(array=w633, length=w627, index=0) -> (deleted portion=w616:string[], array with subset deleted=w618:string[])
        "Result Value" <- w616
        "Saturation_Values" <- w618
        n222 = Build Array(w622, w618) -> (w623:string[][])
        "appended array" <- w623
        n223 = Delete From Array(array=w616, length=4, index=30) -> (deleted portion=w610:string[], array with subset deleted=w614:string[])
        n224 = Search 1D Array(1D array=w610, element="0") -> (index of element=w613:i32)  [unwired: 1 in]
        n225 = disable-structure shown="Enabled" {
          disable-tunnel: [w647 w651] -> w635
          disable-tunnel: w614 -> [w646 w652]
          frame Disabled {
            n226 = Search 1D Array(1D array=w646, element="0") -> (index of element=w650:i32)  [unwired: 1 in]
            n227 = Equal?(x=w650, y=-1) -> (x = y?=w647:bool)
          }
          frame Enabled {
            n228 = for {
              shift-right: [w660] -> _
              shift-left: w652 -> [w662]
              tunnel: [w659] -> w656 mode=indexing if=w657
              tunnel: w652 -> [_] mode=indexing
              stop <- w658 stop-if-true
              n229 = Search 1D Array(1D array=w662, element="0") -> (index of element=w659:i32)  [unwired: 1 in]
              n230 = Less Than 0?(x=w659) -> (x < 0?=w658:bool)
              n231 = Delete From Array(array=w662, length=1, index=w659) -> (array with subset deleted=w660:string[])  [unwired: 1 out]
              n232 = Not(x=w658) -> (.not. x?=w657:bool)
            }
            n233 = Array Size(array=w656) -> (size(s)=w654:i32)
            n234 = Greater?(x=w654, y=2) -> (0:w655:bool)
            n235 = Not(x=w655) -> (.not. x?=w651:bool)
          }
        }
        n236 = Transpose 2D Array(2D array=w623) -> (transposed array=w624:string[][])
        "transposed array" <- w624
        n237 = Equal?(x=w613, y=-1) -> (x = y?=w607:bool)
        n238 = for {
          tunnel: w624 -> [w666] mode=indexing
          tunnel: [w665] -> w625 mode=indexing
          n239 = call <userlib>:"1D Array to String__ogtk.vi"("delimiter (Tab)"="-", "Array of Strings"=w666) -> ("delimited string"=w665:string)  [unwired: 9 in]
        }
        n240 = And(x=w635, y=w607) -> (x .and. y?=w608:bool)
        n241 = call <userlib>:"1D Array to String__ogtk.vi"("delimiter (Tab)"=";", "Array of Strings"=w625) -> ("delimited string"=w617:string)  [unwired: 9 in]
        "Saturation_Values 2" <- w617
        n242 = Select(t=TRUE, s=w608, f=FALSE) -> (s? t:f=w631:bool)
        "Inspection_Result" <- w631
        n243 = Bundle By Name(cluster=T1 {"Inspection_Result 2"=FALSE, "DTU_Inspection_Data"="DTU1_Charge_Percentage,DTU1_Vehicle_Pattern Search,DTU1_R,DTU1_Built_AI OCR,DTU1_Trip_AI OCR,DTU1_1888AI OCR,DTU1_Right_Green_Area,DTU1_Warning,DTU1_Sleep_Mode"} ("Total_Result 2"), "Inspection_Result 2"=w631, "DTU_Inspection_Data"=w617) -> (w634:T1)
        n244 = Bundle By Name(cluster=w641, "Saturation_Values"=w618, "Result Value"=w616, "Total_Result"=w634) -> (w640:T2)
        n245 = case shown="True" w631 {
          tunnel: w629 -> [w670 w675]
          tunnel: [w669 w674] -> w639
          tunnel: w638 -> [_ w673]
          tunnel: w637 -> [w668 _]
          tunnel: w634 -> [_ w672]
          frame False {
            n246 = call-poly "Enqueue Message.vi"("error in (no error)"=w670, "Message"="Failed_Inspections", "Message Queue"=w668) -> ("error out"=w669:errorcluster)  [unwired: 7 in, 1 out]
          }
          frame True {
            n247 = flat-sequence {
              tunnel: w675 -> [w681]
              tunnel: w673 -> [w677]
              tunnel: w672 -> [w676]
              tunnel: [w679] -> w671
              tunnel: [w694] -> w674
              tunnel: w671 -> [w694]
              frame #0 {
                n248 = Unbundle By Name(w681) -> ("status"=w687:bool)
                n249 = call <vilib>:"Clear Errors.vi"("error in (no error)"=w681) -> ("error out"=w680:errorcluster)  [unwired: 5 in, 1 out]
                n250 = Select(t="Error" ("f"), s=w687, f="Read" ("Message")) -> (s? t:f=w683:string)
                n251 = To Variant(anything=w676) -> (Variant=w678:variant)
                n252 = Bundle(cluster=T5 {"Message"="", "Message Data"=variant} ("notification"), "Message"=w683, "Message Data"=w678) -> (w682:T5)
                n253 = Send Notification(notification=w682, notifier=w677, error in (no error)=w680) -> (error out=w679:errorcluster)  [unwired: 1 out]
              }
              frame #1 {
                n254 = Bundle(cluster=T7 {"Status"="", "Free/inuse"=FALSE, "Action"=""} ("Write"), "Status"="FREE" ("Action"), "Free/inuse"=FALSE, "Action"="IDLE" ("Status")) -> (w691:T7)
                n255 = call "FGV_camera_status.vi"("Enum"=enum16{"Init", "Read", "Write"}."Write", "Write"=w691) -> ()  [unwired: 9 in, 1 out]
              }
            }
          }
        }
      }
      frame "Failed_Inspections" {
        w695 = "\n"
        n256 = Unbundle By Name(w712) -> ("DUT"=w708:string, "Result Value"=w727:string[], "notifier out"=w715:refnum<notifier>, "Camera.Prog No."=w701:string)
        n257 = disable-structure shown="Enabled" {
          disable-tunnel: [w757 w758] -> w726
          disable-tunnel: w708 -> [_ w758]
          frame Disabled {
            n258 = local read "Setting Value"() -> (w757:string)
          }
          frame Enabled {
          }
        }
        n259 = Equal?(x=w701, y="9") -> (x = y?=w704:bool)
        n260 = Decimal String To Number(string=w726) -> (number=w725:i32)  [unwired: 2 in, 1 out]
        n261 = case shown="True" w704 {
          tunnel: [w729 w736] -> w703
          tunnel: [w728 w735] -> w702
          tunnel: w701 -> [w732 _]
          frame False {
            n262 = Equal?(x=w732, y="2") -> (x = y?=w730:bool)
            n263 = case shown="True" w730 {
              tunnel: [_ w734] -> w729
              tunnel: [_ w733] -> w728
              frame False {
              }
              frame True {
                n264 = call "Format_DTU_RY.vi"() -> ("DTU2"=w733:string[], "DTU1"=w734:string[])  [unwired: 10 in]
              }
            }
          }
          frame True {
            n265 = call "Format_DTU_RX.vi"() -> ("DTU2"=w735:string[], "DTU1"=w736:string[])  [unwired: 10 in]
          }
        }
        n266 = case shown="2" w725 {
          tunnel: w727 -> [w764 w768]
          tunnel: w703 -> [w763 _]
          tunnel: w702 -> [_ w766]
          tunnel: [w762 w767] -> w722
          tunnel: [w762 w767] -> w718
          frame 1, Default {
            n267 = Build Array(w763, w764) -> (w765:string[][])
            n268 = Transpose 2D Array(2D array=w765) -> (transposed array=w762:string[][])
            "DTU1" <- w762
          }
          frame 2 {
            n269 = Build Array(w766, w768) -> (w769:string[][])
            n270 = Transpose 2D Array(2D array=w769) -> (transposed array=w767:string[][])
            "DTU 2" <- w767
          }
        }
        n271 = Index Array(array=w718, index (col)=1 ("disabled index (col)")) -> (element=w717:string[])  [unwired: 1 in]
        "Result_Values" <- w717
        n272 = local read "Saturation_Values 2"() -> (w696:string)
        n273 = call-poly <userlib>:"Search Array__ogtk.vi"("Array"=w717, "Element Data"="0") -> ("Indices of Elements"=w724:i32[])  [unwired: 7 in]
        "Fail" <- w724
        n274 = Index Array(array=w722, index (col)=0 ("disabled index (col)")) -> (element=w720:string[])  [unwired: 1 in]
        "Inspection_names" <- w720
        n275 = for {
          tunnel: w720 -> [w761]
          tunnel: w724 -> [w760] mode=indexing
          tunnel: [w759] -> w714 mode=indexing
          n276 = Index Array(array=w761, index=w760) -> (element=w759:string)
        }
        "DTU_Failed_Inspections_Array" <- w714
        n277 = Unbundle By Name(w712) -> ("Inspection_Result"=w711:bool)
        n278 = call <userlib>:"1D Array to String__ogtk.vi"("delimiter (Tab)"=";", "Array of Strings"=w714) -> ("delimited string"=w698:string)  [unwired: 9 in]
        "DTU_Failed_Inspections" <- w698
        n279 = Concatenate Strings("Failed Inspections:" ("string"), w695, w698, w695, "Saturation Values:" ("string"), w695, w696) -> (w700:string)
        n280 = Bundle By Name(cluster="Total_Result", "Inspection_Result 2"=w711, "DTU_Inspection_Data"=w700) -> (w710:T1)
        n281 = flat-sequence {
          tunnel: w715 -> [w741]
          tunnel: w706 -> [w740]
          tunnel: w710 -> [w738]
          tunnel: [w739] -> w707
          tunnel: w706 -> [w737]
          tunnel: [w756] -> w713
          tunnel: w707 -> [w756]
          frame #0 {
            n282 = Unbundle By Name(w740) -> ("status"=w749:bool)
            n283 = To Variant(anything=w738) -> (Variant=w742:variant)
            n284 = Select(t="Error" ("f"), s=w749, f="Read" ("Message")) -> (s? t:f=w745:string)
            n285 = Bundle By Name(cluster=T5 {"Message"="", "Message Data"=variant} ("notification"), "Message"=w745, "Message Data"=w742) -> (w744:T5)
            n286 = call <vilib>:"Clear Errors.vi"("error in (no error)"=w737) -> ("error out"=w743:errorcluster)  [unwired: 5 in, 1 out]
            n287 = Send Notification(notification=w744, notifier=w741, error in (no error)=w743) -> (error out=w739:errorcluster)  [unwired: 1 out]
          }
          frame #1 {
            n288 = Bundle(cluster=T7 {"Status"="", "Free/inuse"=FALSE, "Action"=""} ("Write"), "Status"="FREE" ("Action"), "Free/inuse"=FALSE, "Action"="IDLE" ("Status")) -> (w753:T7)
            n289 = call "FGV_camera_status.vi"("Enum"=enum16{"Init", "Read", "Write"}."Write", "Write"=w753) -> ()  [unwired: 9 in, 1 out]
          }
        }
      }
      frame "SSL_Result" {
        n290 = Unbundle By Name(w782) -> ("data out"=w775:string, "notifier out"=w780:refnum<notifier>)  [unwired: 1 out]
        "RX,RY" <- w775
        n291 = Spreadsheet String To Array(delimiter (Tab)="\r", format string="%s", spreadsheet string=w775, array type (2D Dbl)=string[] []) -> (array=w773:string[])
        n292 = Search 1D Array(1D array=w773, element="1") -> (index of element=w771:i32)  [unwired: 1 in]
        n293 = case shown="0, Default" w771 {
          tunnel: ["RX" "RY"] -> w770
          frame 0, Default {
          }
          frame -1 {
          }
        }
        "RX/RY" <- w770
        n294 = flat-sequence {
          tunnel: w780 -> [w789]
          tunnel: w779 -> [w788]
          tunnel: [w787] -> w781
          tunnel: w779 -> [w786]
          tunnel: w770 -> [w785]
          tunnel: [w804] -> w778
          tunnel: w781 -> [w804]
          frame #0 {
            n295 = Unbundle By Name(w788) -> ("status"=w797:bool)
            n296 = To Variant(anything=w785) -> (Variant=w790:variant)
            n297 = Select(t="Error" ("f"), s=w797, f="Read" ("Message")) -> (s? t:f=w793:string)
            n298 = Bundle By Name(cluster=T5 {"Message"="", "Message Data"=variant} ("notification"), "Message"=w793, "Message Data"=w790) -> (w792:T5)
            n299 = call <vilib>:"Clear Errors.vi"("error in (no error)"=w786) -> ("error out"=w791:errorcluster)  [unwired: 5 in, 1 out]
            n300 = Send Notification(notification=w792, notifier=w789, error in (no error)=w791) -> (error out=w787:errorcluster)  [unwired: 1 out]
          }
          frame #1 {
            n301 = Bundle(cluster=T7 {"Status"="", "Free/inuse"=FALSE, "Action"=""} ("Write"), "Status"="FREE" ("Action"), "Free/inuse"=FALSE, "Action"="IDLE" ("Status")) -> (w801:T7)
            n302 = call "FGV_camera_status.vi"("Enum"=enum16{"Init", "Read", "Write"}."Write", "Write"=w801) -> ()  [unwired: 9 in, 1 out]
          }
        }
      }
      frame "Update Display" {
        # "Update Display - Convert the message data to a string to display in the Data Display indicator."
        n303 = Unbundle By Name(w806) -> ("data out"=→"Display <Replace Me>":string)
        n304 = Merge Errors(w807) -> (w808:errorcluster)
      }
      frame "Error" {
        # "#CodeRecommended - If you ever change the name of this \"Error\" message, you'll need to update the name in the Check Loop Error.vi as well."
        # "#CodeRecommended - Consider creating a system for logging errors in some way. These errors are for notification purposes only. Handling of specific errors should be performed in the message frames that generated the error."
        # "Error - Display an error dialog. This message is sent by the \"Error Handler\" VIs at the end of other loops in this application."
        n305 = Variant To Data(error in=w817, type=errorcluster {"status"=FALSE, "code"=0, "source"=""} ("error constant"), Variant=w815) -> (data=w813:errorcluster, error out=w812:errorcluster)
        n306 = call <vilib>:"Simple Error Handler.vi"("error in (no error)"=w813) -> ()  [unwired: 4 in, 5 out]
        n307 = call "FGV_camera_status.vi"("Enum"=enum16{"Init", "Read", "Write"}."Write", "Write"=T7 {"Status"="Error", "Free/inuse"=FALSE, "Action"=""}) -> ()  [unwired: 9 in, 1 out]
        n308 = Merge Errors(w812) -> (w811:errorcluster)
      }
      frame "Reset" {
        # "Reset"
        n309 = call "FGV_camera_status.vi"("Enum"=enum16{"Init", "Read", "Write"}."Write", "Write"=T7 {"Status"="", "Free/inuse"=FALSE, "Action"=""}) -> ()  [unwired: 9 in, 1 out]
        n310 = Merge Errors(w822) -> (w820:errorcluster)
      }
      frame "Confirm Quit" {
        # "Confirm Quit - Message that can confirm whether or not the user wants to exit the application."
        n311 = Unbundle By Name(w823) -> ("notifier out"=w827:refnum<notifier>)
        n312 = Release Notifier(notifier=w827, force destroy? (F)=TRUE, error in (no error)=w825) -> (error out=w824:errorcluster)  [unwired: 2 out]
        n313 = call "Enqueue Message (Single).vi"("Priority Message? (F)"=TRUE, "error in (no error)"=w824, "Message"="Exit", "Message Queue"=w830) -> ("error out"=w831:errorcluster)  [unwired: 6 in, 1 out]
      }
      frame "Exit" {
        # "Stop the VI"
        # "Release the message queue reference"
        # "Exit - Exit the application."
        n314 = Variant To Data(type=errorcluster {"status"=FALSE, "code"=0, "source"=""} ("error constant"), Variant=w839) -> (data=w840:errorcluster)  [unwired: 1 in, 1 out]
        n315 = call <vilib>:"Simple Error Handler.vi"("error in (no error)"=w840) -> ()  [unwired: 4 in, 5 out]
        n316 = Unbundle By Name(w837) -> ("connection ID"=w836:refnum<k5>)
        n317 = TCP Close Connection(connection ID=w836, error in (no error)=w838) -> (error out=w835:errorcluster)  [unwired: 1 in, 1 out]
        n318 = call "Fire User Event - Stop.vi"("User Event - Stop"=w842) -> ("error out"=w833:errorcluster)  [unwired: 10 in]
        n319 = call <vilib>:"Clear Errors.vi"("error in (no error)"=w835) -> ("error out"=w834:errorcluster)  [unwired: 5 in, 1 out]
        n320 = call <vilib>:"Clear Errors.vi"("error in (no error)"=w833) -> ("error out"=w832:errorcluster)  [unwired: 5 in, 1 out]
        n321 = Release Queue(queue=w846, error in (no error)=w834) -> (error out=w844:errorcluster)  [unwired: 1 in, 2 out]
        n322 = Merge Errors(w832, w844) -> (w843:errorcluster)
      }
      frame Default {
        # "'Default' case only runs if there is a message that isn't defined in any of the other cases.  Output a programming error."
        n323 = xnode "Error Ring"("parameter 0"=w847) -> ("error out"=w848:errorcluster)
      }
    }
    n324 = call "Error Handler - Message Handling Loop.vi"("error in (no error)"=w24, "Message Queue"=w26) -> ("dup error in"=w25:errorcluster)  [unwired: 8 in, 1 out]
  }
  n325 = while {
    tunnel: w5 -> [w863]
    shift-right: [w861] -> w18
    shift-left: w15 -> [w862]
    tunnel: [w857] -> w16
    stop <- w859 stop-if-true
    # "Event Handling Loop"
    n326 = event shown="[5] \"Change_Program\": Value Change" {
      selector: w862 -> [_ _ _ _ _ _]
      dyn-events: [_ _ _ _ _ _] -> w861
      timeout: _ -> [_ _ _ _ _ _]
      tunnel: [_ _ _ TRUE ("Discard?") _ _] -> w859
      tunnel: w863 -> [w868 w870 w875 w878 w882 w886]
      tunnel: [w867 _ w874 _ w879 w885] -> w860
      tunnel: [w866 w870 w873 w878 w881 w884] -> w858
      event Panel Close? {
        # "Send the 'Confirm Quit' message if the user closes the panel of the VI. Discard the event so the 'Confirm Quit' message has a chance to run."
        n327 = event-data() -> ()  [unwired: 1 in, 1 out]
        n328 = call "Enqueue Message (Single).vi"("Priority Message? (F)"=TRUE, "Message"="Confirm Quit", "Message Queue"=w868) -> ("error out"=w867:errorcluster, "dup Message Queue"=w866:refnum<queue>)  [unwired: 7 in]
        n329 = event-data("Discard?"=TRUE) -> ()  [unwired: 1 in, 1 out]
      }
      event Application Instance Close {
        # "#CodeRecommended - When a project closes, all VIs within that project are aborted and leave memory. However, any code placed in this event frame is guaranteed to run to completion, so add any cleanup code that absolutely must happen here."
        n330 = event-data() -> ()  [unwired: 1 in, 1 out]
      }
      event "Exit": Value Change {
        n331 = event-data() -> ()  [unwired: 1 in, 1 out]
        n332 = call "Enqueue Message (Single).vi"("Priority Message? (F)"=TRUE, "Message"="Exit", "Message Queue"=w875) -> ("error out"=w874:errorcluster, "dup Message Queue"=w873:refnum<queue>)  [unwired: 7 in]
      }
      event User Event {
        # "The Message Handling Loop processed an \"Exit\" message, which fired this event to stop the Event Handling Loop."
        n333 = event-data() -> ()  [unwired: 1 in, 1 out]
        n334 = local write "Display <Replace Me>"("\"Exit\" button pressed" ("VI Stopped")) -> ()
      }
      event "Trigger": Value Change {
        n335 = event-data() -> ()  [unwired: 1 in, 1 out]
        n336 = call "Enqueue Message (Single).vi"("Message"="Trigger", "Message Queue"=w882) -> ("error out"=w879:errorcluster, "dup Message Queue"=w881:refnum<queue>)  [unwired: 8 in]
      }
      event "Change_Program": Value Change {
        n337 = event-data() -> ()  [unwired: 1 in, 1 out]
        n338 = call "Enqueue Message (Single).vi"("Message"="Change_Program", "Message Queue"=w886) -> ("error out"=w885:errorcluster, "dup Message Queue"=w884:refnum<queue>)  [unwired: 8 in]
      }
    }
    n339 = call "Error Handler - Event Handling Loop.vi"("error in (no error)"=w860, "Message Queue"=w858) -> ("dup error in"=w857:errorcluster)  [unwired: 8 in, 1 out]
  }
  n340 = Unregister For Events(event registration refnum=w18, error in=w16) -> (error out=w19:errorcluster)
  n341 = Merge Errors(w19, w22) -> (w20:errorcluster)
  n342 = call "Destroy User Event - Stop.vi"("error in (no error)"=w20, "User Event - Stop"=w14) -> ("error out"=w17:errorcluster)  [unwired: 9 in]
  n343 = disable-structure shown="Default" {
    disable-tunnel: w17 -> [_ _]
    frame condition #0 (active) {
    }
    frame condition #1 {
      # "Call Quit LabVIEW if running as a built application."
      n344 = Quit LabVIEW() -> ()  [unwired: 1 in]
    }
  }
